vi "Test Load Instruments.vi"(11 "Test Case In":refnum<class "Test Instrument Manager AE.lvclass">) -> (0 "error out":errorcluster, 3 "Test Case Out":refnum<class "Test Instrument Manager AE.lvclass">)   [LabVIEW 2020, in "Test Instrument Manager AE.lvclass"]
uses:
  Test Instrument Manager AE.lvclass
  C:/Program Files/National Instruments/LabVIEW 2025/vi.lib/Astemes/LUnit/Test Case.lvclass
  <vilib>/Astemes/LUnit/Test Case.lvclass/Test Case.ctl
  Test Instrument Manager AE.lvclass/Test Instrument Manager AE.ctl
  4993e8ee-a06a-463a-9684-69129f64d5ce.vi
  Source/Instrument Manager AE/Instrument Manager AE.lvlib
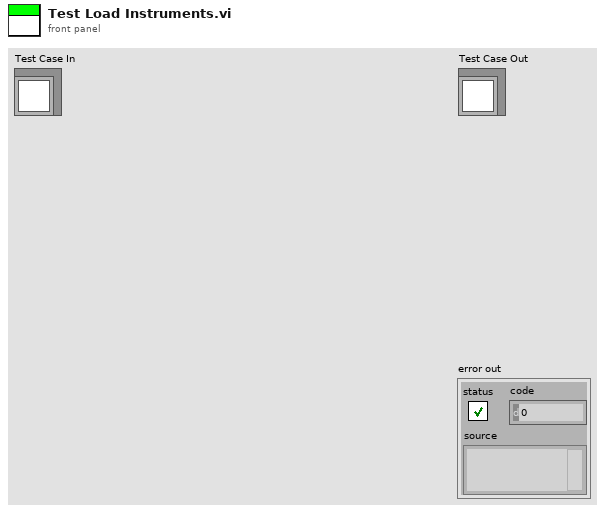
[diagram p1: front panel]
types:
  T1 = enum16{"Close", "Close Instrument", "Load Instruments", "Get Instrument"}
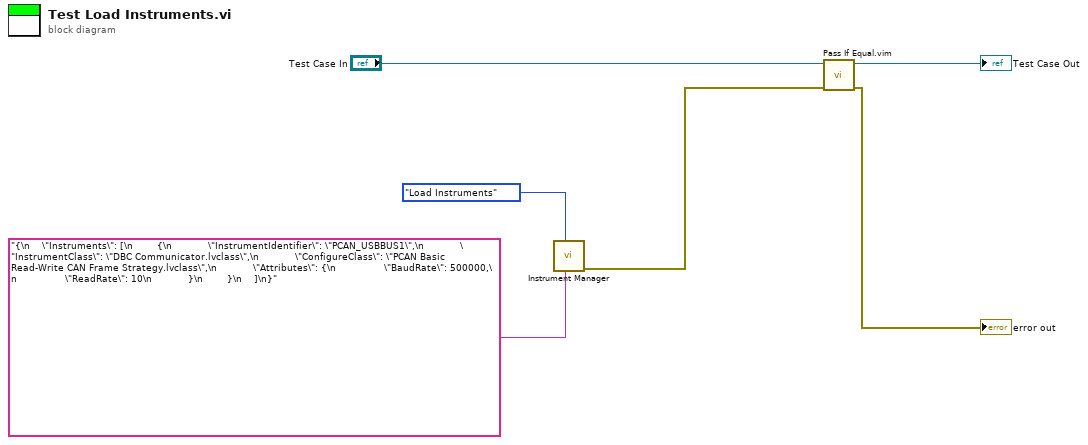
[diagram p0: block diagram]
diagram:
  n1 = call "Instrument Manager.vi"("Source"="{\n    \"Instruments\": [\n        {\n            \"InstrumentIdentifier\": \"PCAN_USBBUS1\",\n            \"InstrumentClass\": \"DBC Communicator.lvclass\",\n            \"ConfigureClass\": \"PCAN Basic Read-Write CAN Frame Strategy.lvclass\",\n            \"Attributes\": {\n                \"BaudRate\": 500000,\n                \"ReadRate\": 10\n            }\n        }\n    ]\n}", "Operation"=T1."Load Instruments") -> ("error out"=w1:errorcluster)  [unwired: 9 in]
  n2 = call "Pass If Equal.vim"("error in (no error)"=w1, "LUnit Test Case In"="Test Case In") -> ("error out"=→"error out":errorcluster, "LUnit Test Case Out"=→"Test Case Out":refnum<class "Test Instrument Manager AE.lvclass">)  [unwired: 8 in]
